vi "p4.1.vi"() -> ()   [LabVIEW 2020]
uses:
  <vilib>/Analysis/2dsp.llb/Decimate (continuous, DBL).vi
  <vilib>/Analysis/NI_AALBase.lvlib
  <vilib>/Analysis/NI_AALPro.lvlib
panel:
  out "FFT(Diezmado M=3)":dbl[](graph)
  out "FFT(Diezmado M=2)":dbl[](graph)
  out "FFT(original)":dbl[](graph)
  in  "M =3":i32=1
  out "Diezmado M=3":dbl[](graph)
  out "Diezmado M=2":dbl[](graph)
  in  "M=2":i32=1
  out "cos(0,2pi) + cos(0,3pi) - Original":dbl[](graph)
  in  "Frecuencia cos(0,3pi)":dbl=0.0078125 format="%0.4e"
  out "cos(0,3pi)":dbl[](graph)
  out "cos(0,2pi)":dbl[](graph)
  in  "Frecuencia cos(0,2pi)":dbl=0.0078125 format="%0.4e"
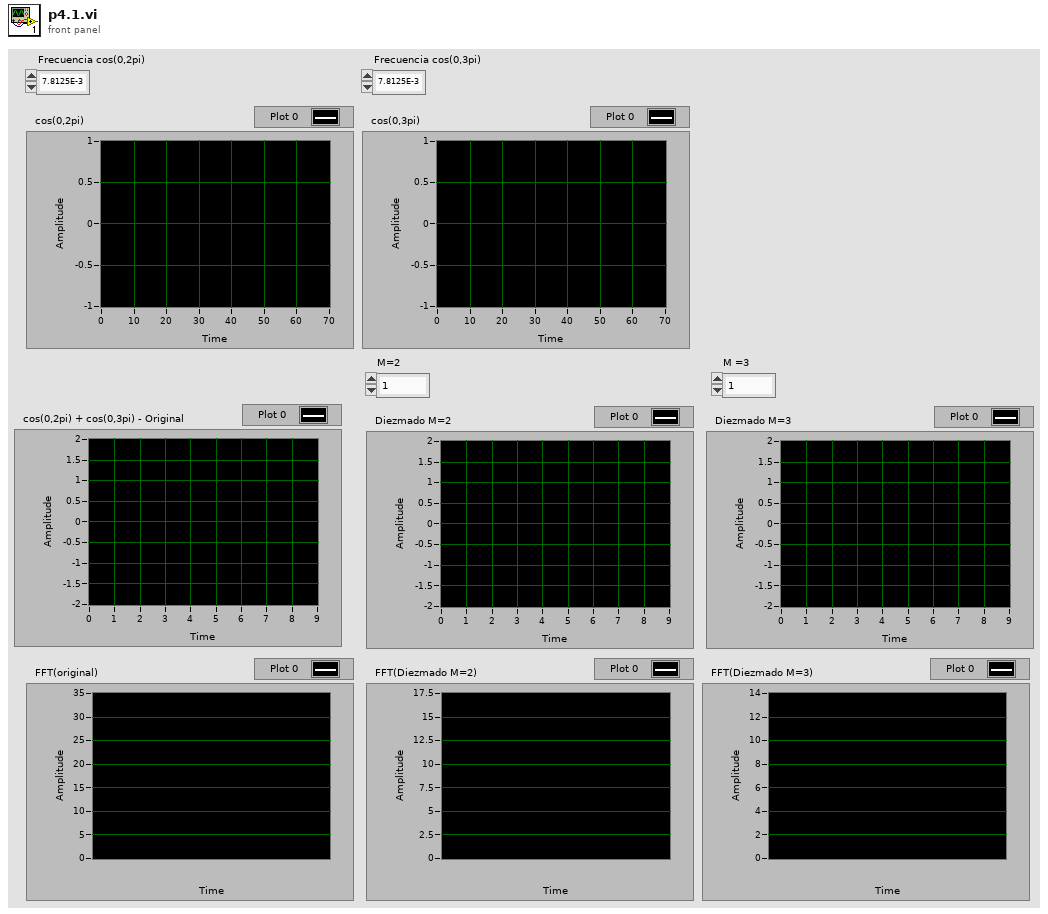
[diagram p1: front panel]
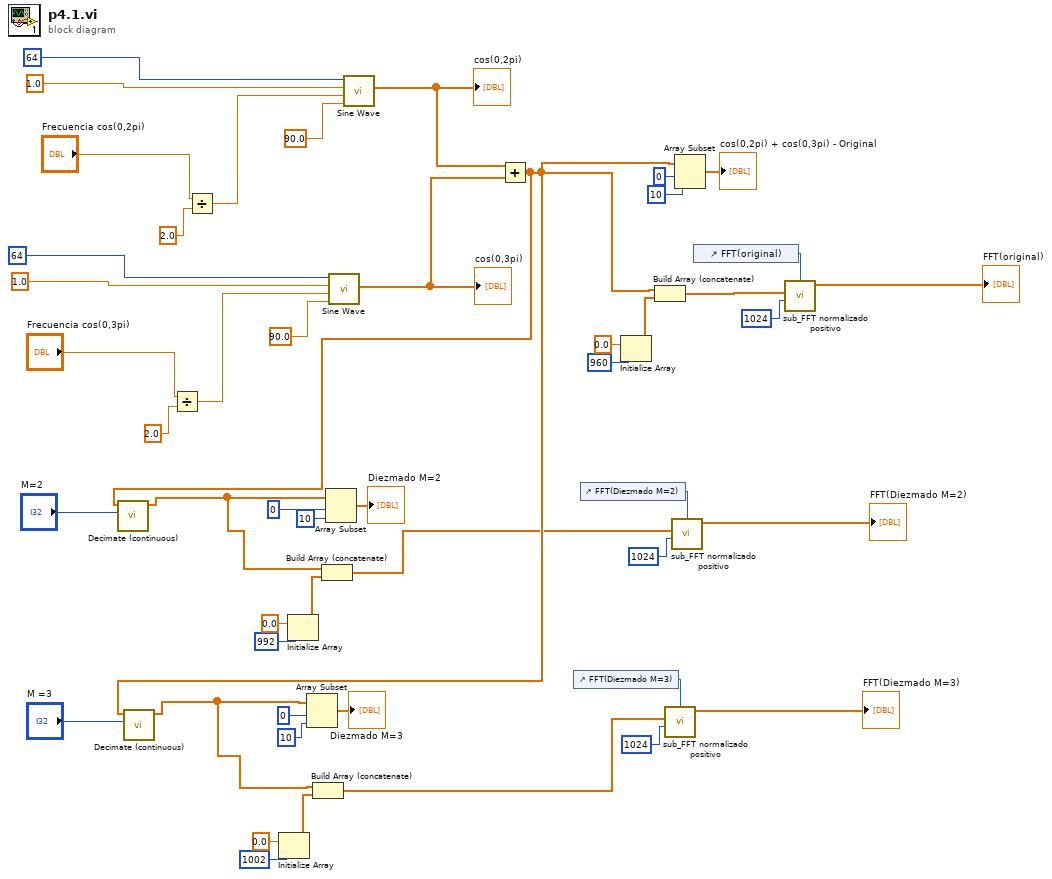
[diagram p0: block diagram]
diagram:
  n1 = Divide(x="Frecuencia cos(0,3pi)", y=2.0) -> (x/y=w42:dbl)
  n2 = Divide(x="Frecuencia cos(0,2pi)", y=2.0) -> (x/y=w45:dbl)
  n3 = Initialize Array(0.0 ("element"), 1002 ("dimension size")) -> (w5:dbl[])
  n4 = Initialize Array(0.0 ("element"), 992 ("dimension size")) -> (w10:dbl[])
  n5 = call <vilib>:"Sine Wave.vi"("samples"=64, "amplitude"=1.0, "frequency"=w42, "phase in"=90.0) -> ("sine wave"=w36:dbl[])  [unwired: 1 in, 2 out]
  "cos(0,3pi)" <- w36
  n6 = call <vilib>:"Sine Wave.vi"("samples"=64, "amplitude"=1.0, "frequency"=w45, "phase in"=90.0) -> ("sine wave"=w37:dbl[])  [unwired: 1 in, 2 out]
  "cos(0,2pi)" <- w37
  n7 = Add(x=w37, y=w36) -> (x+y=w22:dbl[])
  n8 = call-poly <vilib>:"Decimate (continuous).vi"("decimating factor"="M=2", "X"=w22) -> ("Decimated Array"=w4:dbl[])  [unwired: 8 in, 1 out]
  n9 = call-poly <vilib>:"Decimate (continuous).vi"("decimating factor"="M =3", "X"=w22) -> ("Decimated Array"=w3:dbl[])  [unwired: 8 in, 1 out]
  n10 = Array Subset(array=w3, index=0, length=10) -> (→"Diezmado M=3":dbl[])
  n11 = Build Array (concatenate)(w3, w5) -> (w2:dbl[])
  n12 = Build Array (concatenate)(w4, w10) -> (w1:dbl[])
  n13 = Array Subset(array=w4, index=0, length=10) -> (→"Diezmado M=2":dbl[])
  n14 = control-ref of="FFT(Diezmado M=3)"() -> (w11:refnum<vi>)
  n15 = control-ref of="FFT(Diezmado M=2)"() -> (w16:refnum<vi>)
  n16 = Initialize Array(0.0 ("element"), 960 ("dimension size")) -> (w19:dbl[])
  n17 = Build Array (concatenate)(w22, w19) -> (w18:dbl[])
  n18 = call "sub_FFT normalizado positivo.vi"("FFT size"=1024, "Array in"=w2, "WaveformGraph in"=w11) -> ("Array out"=→"FFT(Diezmado M=3)":dbl[])  [unwired: 8 in]
  n19 = call "sub_FFT normalizado positivo.vi"("FFT size"=1024, "Array in"=w1, "WaveformGraph in"=w16) -> ("Array out"=→"FFT(Diezmado M=2)":dbl[])  [unwired: 8 in]
  n20 = Array Subset(array=w22, index=0, length=10) -> (→"cos(0,2pi) + cos(0,3pi) - Original":dbl[])
  n21 = control-ref of="FFT(original)"() -> (w17:refnum<vi>)
  n22 = call "sub_FFT normalizado positivo.vi"("FFT size"=1024, "Array in"=w18, "WaveformGraph in"=w17) -> ("Array out"=→"FFT(original)":dbl[])  [unwired: 8 in]
